vi "Set Unit ID.vi"(8 "error in (no error)":errorcluster, 10 "Unit ID":u8, 11 "Modbus master in":refnum<class "Network Master.lvclass">) -> (0 "error out":errorcluster, 3 "Modbus master out":refnum<class "Network Master.lvclass">)   [LabVIEW 2021, in "Network Master.lvclass"]
doc: "<B>Unit ID</B> specifies the identification of a serial Modbus slave. You can use a Modbus master instance to perform read and write operations on this Modbus slave. The Property Node ignores requests from TCP Modbus master instances."
uses:
  Network Master.lvclass
  Network Master.lvclass/Network Master.ctl
  Transmission Data Unit/Transmission Data Unit.lvclass/Transmission Data Unit.ctl
  Transmission Data Unit/Transmission Data Unit.lvclass
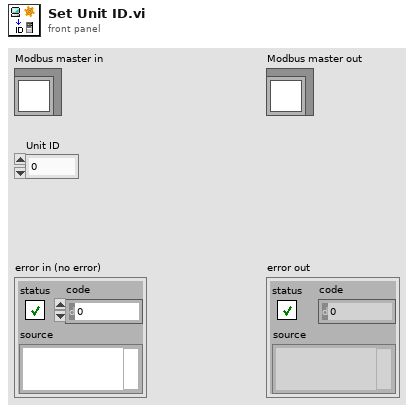
[diagram p1: front panel]
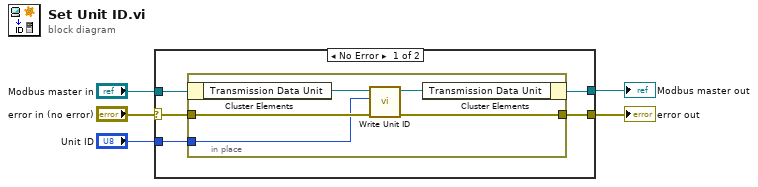
[diagram p0: block diagram]
diagram:
  n1 = case shown="No Error" "error in (no error)" {
    selector: "error in (no error)" -> [w8 w16]
    tunnel: "Unit ID" -> [w6 _]
    tunnel: [w9 w17] -> w2
    tunnel: "Modbus master in" -> [w10 w17]
    tunnel: [w7 w16] -> w1
    frame No Error {
      n2 = in-place {
        in-place-border: w8 -> [w12]
        in-place-border: [w15] -> w7
        in-place-border: w6 -> [w11]
        n3 = in-place-cluster #1(w10) -> ("Transmission Data Unit"=w13:refnum<class "Transmission Data Unit.lvclass">)
        n4 = call "Write Unit ID.vi"("error in"=w12, "unit ID"=w11, "transmission data unit in"=w13) -> ("error out"=w15:errorcluster, "transmission data unit out"=w14:refnum<class "Transmission Data Unit.lvclass">)  [unwired: 7 in]
        n5 = in-place-cluster #1("Transmission Data Unit"=w14) -> (w9:refnum<class "Network Master.lvclass">)
      }
    }
    frame Error {
    }
  }
  "error out" <- w1
  "Modbus master out" <- w2
